vi "start.vi"(8 "error in (no error)":errorcluster, 11 "Pixelfly in":refnum<class "Pixelfly.lvclass">) -> (0 "error out":errorcluster, 3 "Pixelfly out":refnum<class "Pixelfly.lvclass">)   [LabVIEW 2009, in "Hardware.lvlib" / "Channels.lvlib" / "Pixelfly.lvclass"]
uses:
  Pixelfly.lvclass
  Tools/CameraSettings/PixelFlySettings/PixelflySettings.lvclass
  Pixelfly.lvclass/Pixelfly.ctl
  Camera.lvclass
  Channels.lvlib
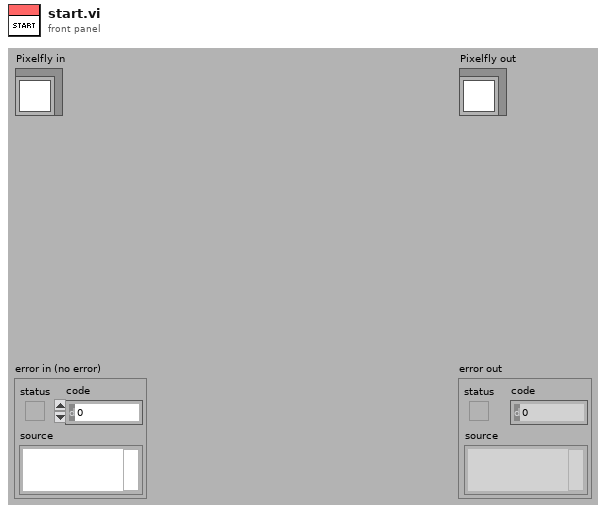
[diagram p1: front panel]
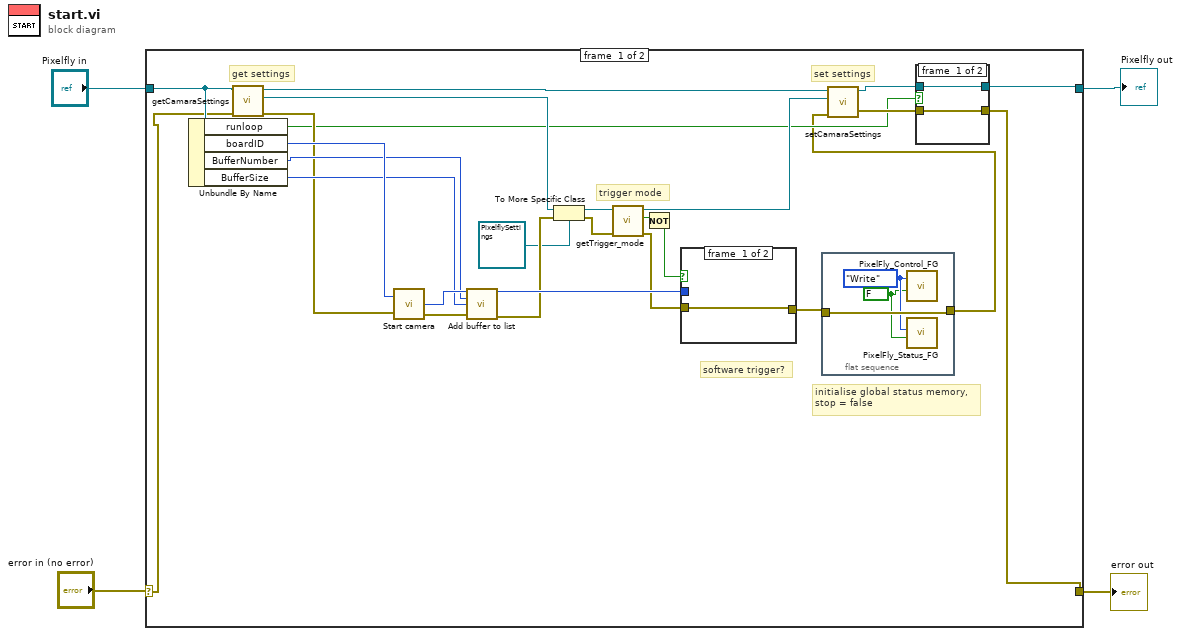
[diagram p0: block diagram]
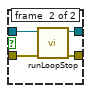
[diagram p2: hidden frame]
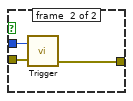
[diagram p3: hidden frame]
diagram:
  n1 = case shown="No Error" "error in (no error)" {
    selector: "error in (no error)" -> [w23 w44]
    tunnel: [w8 w44] -> w3
    tunnel: [w9 w45] -> w2
    tunnel: "Pixelfly in" -> [w24 w45]
    frame #0 {
      # "initialise global status memory,\nstop = false"
      # "set settings"
      # "get settings"
      # "trigger mode"
      # "software trigger?"
      n2 = Unbundle By Name(w24) -> ("runloop"=w7:bool, "boardID"=w27:i32, "BufferNumber"=w26:i32, "BufferSize"=w25:i32)
      n3 = call "getCamaraSettings.vi"("error in (no error)"=w23, "Camera in"=w24) -> ("error out"=w22:errorcluster, "CamaraSettings"=w21:refnum<class "CamaraSettings.lvclass">, "Camera out"=w13:refnum<class "Pixelfly.lvclass">)  [unwired: 7 in]
      n4 = call <instrlib>:"Start camera.vi"("Handle in"=w27, "error in (no error)"=w22) -> ("Handle out"=w30:i32, "error out"=w29:errorcluster)  [unwired: 1 out]
      n5 = call <instrlib>:"Add buffer to list.vi"("Handle in"=w30, "Buffer in"=w26, "size"=w25, "error in (no error)"=w29) -> ("Handle out"=w28:i32, "error out"=w20:errorcluster)  [unwired: 9 in, 1 out]
      n6 = To More Specific Class(target class=refnum<class "PixelflySettings.lvclass"> refnum ("Tools.lvlib:Settings.lvlib:PixelflySettings.lvclass"), reference=w21, error in=w20) -> (specific class reference=w19:refnum<class "PixelflySettings.lvclass">, error out=w18:errorcluster)
      n7 = call "getTrigger_mode.vi"("error in (no error)"=w18, "PixelflySettings in"=w19) -> ("error out"=w16:errorcluster, "trigger_mode"=w15:bool, "PixelflySettings out"=w12:refnum<class "PixelflySettings.lvclass">)  [unwired: 7 in]
      n8 = Not(x=w15) -> (.not. x?=w14:bool)
      n9 = case shown="False" w14 {
        tunnel: w28 -> [_ w43]
        tunnel: w16 -> [w40 w42]
        tunnel: [w40 w41] -> w6
        frame #0 {
        }
        frame #1 {
          n10 = call <instrlib>:"Trigger.vi"("Handle in"=w43, "error in (no error)"=w42) -> ("error out"=w41:errorcluster)  [unwired: 2 out]
        }
      }
      n11 = flat-sequence {
        tunnel: [w33] -> w5
        tunnel: w6 -> [w33]
        frame #0 {
          w32 = enum16{"Write", "Read"}."Write" ("Action")
          w31 = FALSE
          n12 = call "PixelFly_Control_FG.vi"("stop"=w31, "Action"=w32) -> ()  [unwired: 9 in, 1 out]
          n13 = call "PixelFly_Status_FG.vi"("stop"=w31, "Action"=w32) -> ()  [unwired: 9 in, 1 out]
        }
      }
      n14 = call "setCamaraSettings.vi"("error in (no error)"=w5, "CamaraSettings"=w12, "Camera in"=w13) -> ("error out"=w10:errorcluster, "Camera out"=w11:refnum<class "Pixelfly.lvclass">)  [unwired: 7 in]
      n15 = case shown="True" w7 {
        tunnel: w11 -> [w35 w39]
        tunnel: w10 -> [w34 w38]
        tunnel: [w35 w37] -> w9
        tunnel: [w34 w36] -> w8
        frame #0 {
        }
        frame #1 {
          n16 = call "runLoopStop.vi"("error in (no error)"=w38, "Pixelfly in"=w39) -> ("error out"=w36:errorcluster, "Pixelfly out"=w37:refnum<class "Pixelfly.lvclass">)  [unwired: 8 in]
        }
      }
    }
    frame #1 {
    }
  }
  "error out" <- w3
  "Pixelfly out" <- w2
